vi "Kronecker Product.vi"   [LabVIEW 2020, in "NI_AALPro.lvlib"]
doc: "Calculates the Kronecker product of the input matrices <B>A</B> and <B>B</B>. The data types you wire to the <B>A</B> and <B>B</B> inputs determine the polymorphic instance to use."
uses:
  <vilib>/Analysis/NI_AALPro.lvlib
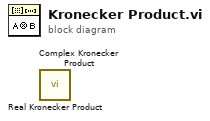
[diagram p0: block diagram]
diagram:
  n1 = call <vilib>:"Real Kronecker Product.vi"() -> ()  [unwired: 10 in, 2 out]
  n2 = call <vilib>:"Complex Kronecker Product.vi"() -> ()  [unwired: 10 in, 2 out]
